vi "Mouse Move Event.vi"(8 "错误输入（无错误）":errorcluster, 10 "Mode":enum16{"Absolute", "Relative"}(ring), 11 "Position":cluster{"dx":u32, "dy":u32}) -> (0 "错误输出":errorcluster)   [LabVIEW 2012, in "API.lvlib"]
uses:
  API.lvlib
  Mouse_Event.ctl
  user32.dll
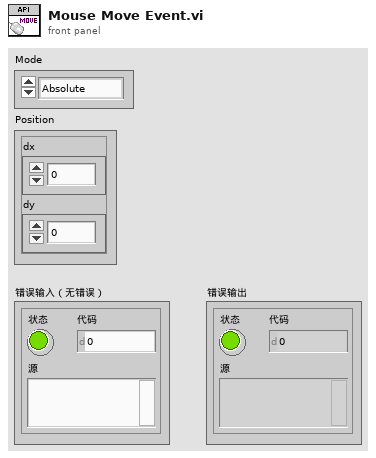
[diagram p1: front panel]
types:
  T1 = typedef "API.lvlib/Mouse_Event.ctl" = u32
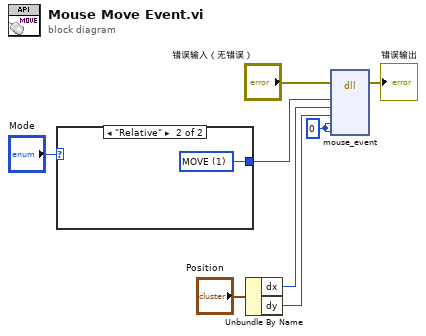
[diagram p0: block diagram]
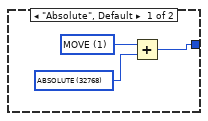
[diagram p2: hidden frame]
diagram:
  w3 = u32 0 ("dwExtraInfo")
  n1 = case shown="\"Relative\"" "Mode" {
    tunnel: [w9 w12] -> w7
    frame "Absolute", Default {
      w10 = T1 32768 items=["MOVE"=1, "LEFT_DOWN"=2, "lEFT_UP"=4, "RIGHT_DOWN"=8, "RIGHT_UP"=16, "MIDDLE_DOWN"=32, "MIDDLE_UP"=64, "MOUSE_WHEEL"=128, "ABSOLUTE"=32768] ("文本下拉列表")
      w11 = T1 1 items=["MOVE"=1, "LEFT_DOWN"=2, "lEFT_UP"=4, "RIGHT_DOWN"=8, "RIGHT_UP"=16, "MIDDLE_DOWN"=32, "MIDDLE_UP"=64, "MOUSE_WHEEL"=128, "ABSOLUTE"=32768] ("文本下拉列表")
      n2 = Add(x=w11, y=w10) -> (x+y=w9:T1)
    }
    frame "Relative" {
      w12 = T1 1 items=["MOVE"=1, "LEFT_DOWN"=2, "lEFT_UP"=4, "RIGHT_DOWN"=8, "RIGHT_UP"=16, "MIDDLE_DOWN"=32, "MIDDLE_UP"=64, "MOUSE_WHEEL"=128, "ABSOLUTE"=32768] ("文本下拉列表")
    }
  }
  n3 = Unbundle By Name("Position") -> ("dx"=w5:u32, "dy"=w4:u32)
  n4 = dll-call lib="user32.dll" fn="mouse_event"(error in="错误输入（无错误）", "dwFlags"=w7, "dx"=w5, "dy"=w4, "dwData"=w3, "dwExtraInfo"=w3) -> (error out=→"错误输出":errorcluster)  [unwired: 8 in, 1 out]
